vi "rqp_Start Exiting.vi"(7 "Caller in":refnum<class "Worker.lvclass">, 8 "error in":errorcluster, 11 "DMM HAL in":refnum<class "Interface 1.lvclass">) -> (0 "error out":errorcluster, 3 "dup DMM HAL out":refnum<class "Interface 1.lvclass">)   [LabVIEW 2020, in "Interface 1.lvclass"]
doc: "This VI will indirectly send a message to the <Start Exiting> MHL case of the Worker that own this VI.\n---\nThe shutdown sequence of the Worker that owns this VI will be initiated."
uses:
  Interface 1.lvclass
  <vilib>/addons/_Workers/Library/Classes/Worker/Worker.lvclass
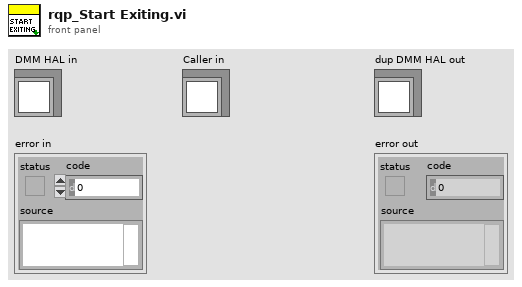
[diagram p1: front panel]
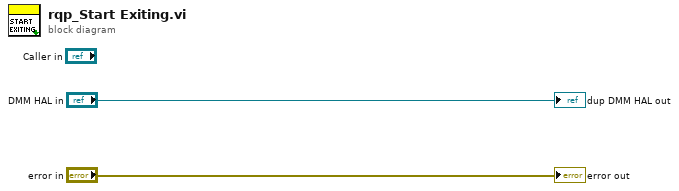
[diagram p0: block diagram]
diagram:
  "error out" <- "error in"
  "dup DMM HAL out" <- "DMM HAL in"
